vi "Convert Variant to Data String.vi"(8 "error in (no error)":errorcluster, 11 "Data Value":variant) -> (0 "error out":errorcluster, 2 "Data Value String":string)   [LabVIEW 2016, in "Assert API Components.lvlib" / "Assert Display.lvlib"]
doc: "Converts a variant piece of data to a string via the correct data type for the data contained in the variant"
uses:
  Assert Display.lvlib
  <vilib>/Utility/Data Type/NI_Data Type.lvlib
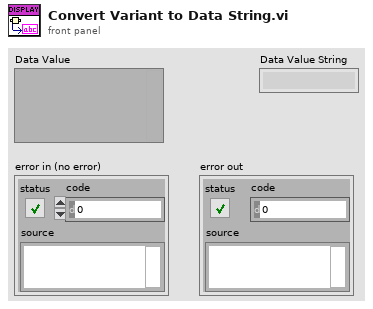
[diagram p1: front panel]
types:
  T1 = typedef "NI_Data Type.lvlib/Data Type.ctl" = enum8{"Invalid Type", "Void", "I8", "I16", "I32", "I64", "U8", "U16", "U32", "U64", "Single Float", "Double Float", "Extended Float", "Single Complex", "Double Complex", "Extended Complex", "Enum U8", "Enum U16", "Enum U32", "Enum U64", "Single Float With Unit", "Double Float With Unit", "Extended Float With Unit", "Single Complex with Unit", "Double Complex with Unit", "Extended Complex with Unit", "Boolean", "String", "Path", "Picture", "Tag", "Array", "Cluster", "Variant", "LV Variant", "Waveform", "Timestamp", "Digital Waveform", "Digital Data", "ExpressData", "Refnum", "External Data", "VI", "Poly VI", "LabVIEW Class Instance", "Fixed Point"}
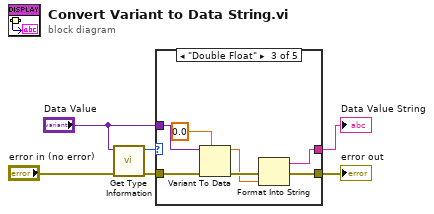
[diagram p0: block diagram]
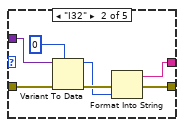
[diagram p3: hidden frame]
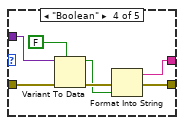
[diagram p4: hidden frame]
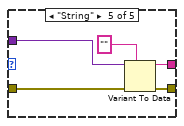
[diagram p5: hidden frame]
diagram:
  n1 = call <vilib>:"Get Type Information.vi"("error in (no error)"="error in (no error)", "Variant"="Data Value") -> ("error out"=w3:errorcluster, "Type"=w1:T1)  [unwired: 5 in, 3 out]
  n2 = case shown="\"Double Float\"" w1 {
    tunnel: [w7 w14 w21 w28 w33] -> w6
    tunnel: [_ w12 w19 w26 w32] -> w5
    tunnel: w3 -> [w7 w9 w16 w23 w30]
    tunnel: "Data Value" -> [_ w8 w15 w22 w29]
    frame "Invalid Type", Default {
    }
    frame "I32" {
      n3 = Variant To Data(error in=w9, type=0, Variant=w8) -> (data=w11:i32, error out=w13:errorcluster)
      n4 = Format Into String(error in=w13, w11) -> (resulting string=w12:string, error out=w14:errorcluster)  [unwired: 2 in]
    }
    frame "Double Float" {
      n5 = Variant To Data(error in=w16, type=0.0, Variant=w15) -> (data=w18:dbl, error out=w20:errorcluster)
      n6 = Format Into String(error in=w20, w18) -> (resulting string=w19:string, error out=w21:errorcluster)  [unwired: 2 in]
    }
    frame "Boolean" {
      n7 = Variant To Data(error in=w23, type=FALSE, Variant=w22) -> (data=w25:bool, error out=w27:errorcluster)
      n8 = Format Into String(error in=w27, w25) -> (resulting string=w26:string, error out=w28:errorcluster)  [unwired: 2 in]
    }
    frame "String" {
      n9 = Variant To Data(error in=w30, type="", Variant=w29) -> (data=w32:string, error out=w33:errorcluster)
    }
  }
  "error out" <- w6
  "Data Value String" <- w5
